vi "MainControlPanel.vi"() -> ()   [LabVIEW 2016]
uses:
  GlobalControlVariables.vi
panel:
  out "Owned":bool
  in  "Acquire Sema":bool
  out "Sema Avail":dbl
  out "Timed Out Sema":bool
  out "Error Messages":string
  in  "QuitVI":bool
  in  "Disconnect":bool
  in  "Chassis Port":u16=8088
  in  "Open Module\n   Controller:":bool
  in  "Module Slot":string(combo)="1"
  out "Connected?":bool
  in  "Connect":bool
  in  "Chassis Address":string="127.0.0.1"
  in  "Module Type":string(combo)="NI-9218"
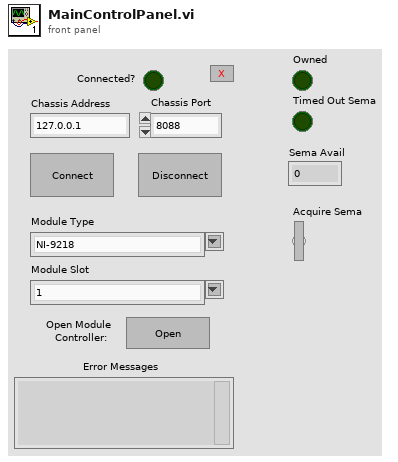
[diagram p1: front panel]
types:
  T1 = typedef "Semaphore RefNum" = refnum<k1>
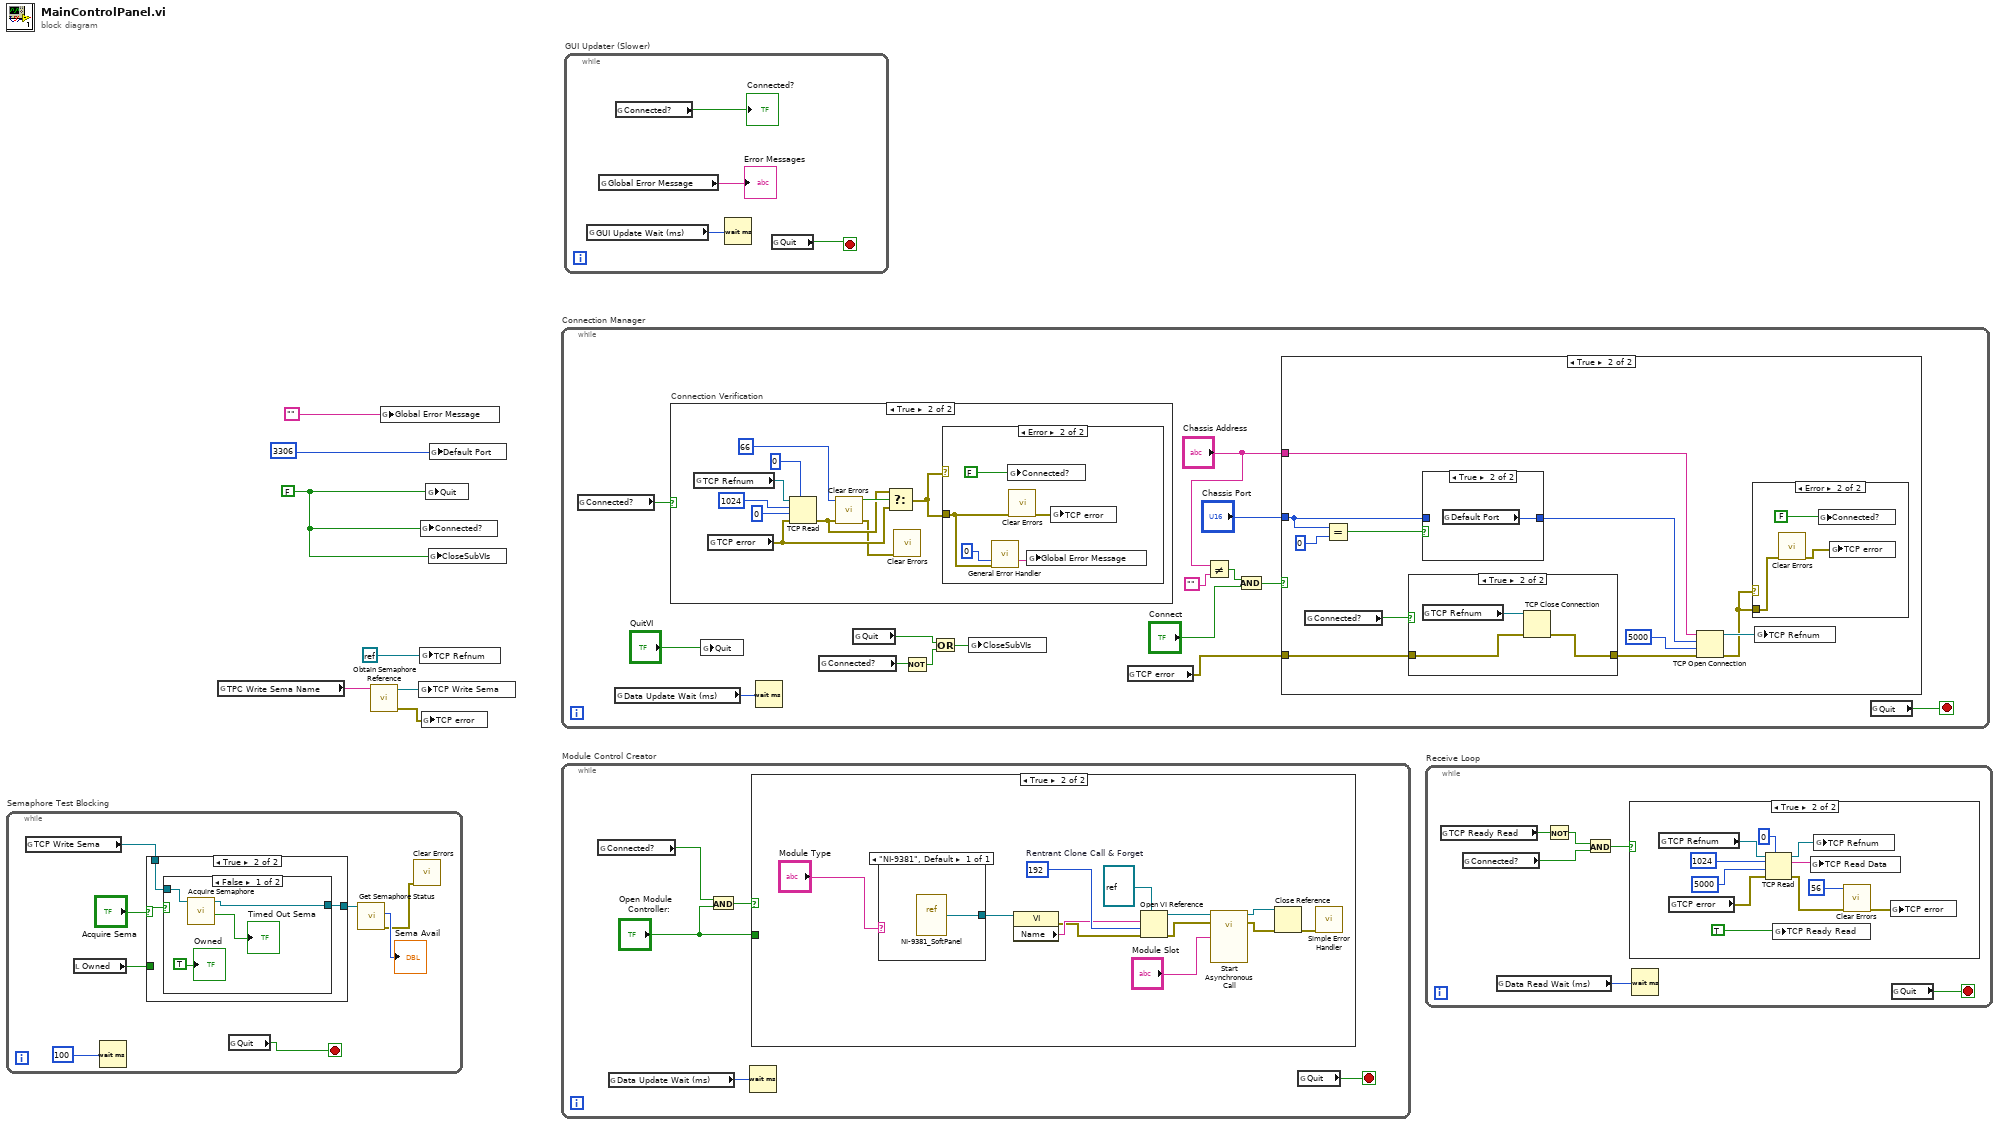
[diagram p0: block diagram]
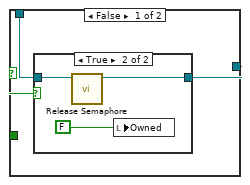
[diagram p2: hidden frame]
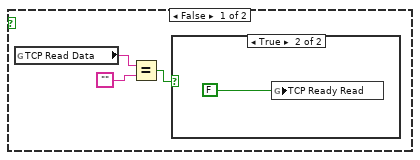
[diagram p5: hidden frame]
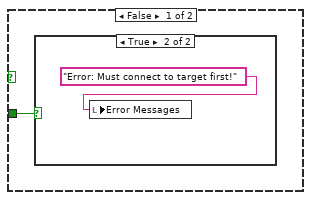
[diagram p7: hidden frame]
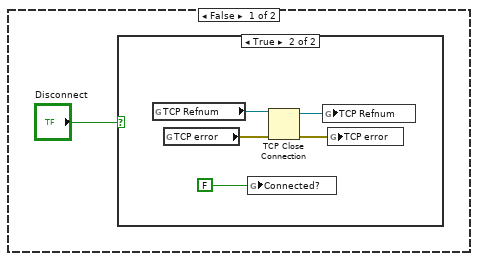
[diagram p11: hidden frame]
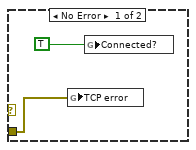
[diagram p13: hidden frame]
diagram:
  w1 = FALSE
  n1 = while "Semaphore Test Blocking" {
    stop <- w14 stop-if-true
    n2 = global read "GlobalControlVariables.vi" "TCP Write Sema"() -> (w9:T1)
    n3 = local read "Owned"() -> (w10:bool)
    n4 = Wait (ms)(milliseconds to wait=u32 100) -> ()  [unwired: 1 out]
    n5 = case shown="True" "Acquire Sema" {
      tunnel: [w18 w25] -> w13
      tunnel: w10 -> [w17 w24]
      tunnel: w9 -> [w16 w23]
      frame False {
        n6 = case shown="True" w17 {
          tunnel: w16 -> [w19 w22]
          tunnel: [w19 w21] -> w18
          frame False {
          }
          frame True {
            n7 = call <vilib>:"Release Semaphore.vi"("semaphore"=w22) -> ("semaphore out"=w21:T1)  [unwired: 5 in, 1 out]
            n8 = local write "Owned"(FALSE) -> ()
          }
        }
      }
      frame True {
        n9 = case shown="False" w24 {
          tunnel: w23 -> [w29 w30]
          tunnel: [w28 w30] -> w25
          frame False {
            n10 = call <vilib>:"Acquire Semaphore.vi"("semaphore"=w29) -> ("timed out"=→"Timed Out Sema":bool, "semaphore out"=w28:T1)  [unwired: 4 in, 1 out]
            "Owned" <- TRUE
          }
          frame True {
          }
        }
      }
    }
    n11 = global read "GlobalControlVariables.vi" "Quit"() -> (w14:bool)
    n12 = call <vilib>:"Get Semaphore Status.vi"("semaphore"=w13) -> ("error out"=w8:errorcluster, "# available"=→"Sema Avail":i32)  [unwired: 5 in, 4 out]
    n13 = call <vilib>:"Clear Errors.vi"("error in (no error)"=w8) -> ()  [unwired: 5 in, 2 out]
  }
  n14 = global read "GlobalControlVariables.vi" "TPC Write Sema Name"() -> (w4:string)
  n15 = call <vilib>:"Obtain Semaphore Reference.vi"("name (unnamed)"=w4) -> ("error out"=w2:errorcluster, "semaphore"=w3:T1)  [unwired: 4 in, 1 out]
  n16 = global write "GlobalControlVariables.vi" "Global Error Message"("") -> ()
  n17 = global write "GlobalControlVariables.vi" "TCP Write Sema"(w3) -> ()
  n18 = global write "GlobalControlVariables.vi" "TCP Refnum"(refnum<k0> refnum) -> ()
  n19 = global write "GlobalControlVariables.vi" "Connected?"(w1) -> ()
  n20 = global write "GlobalControlVariables.vi" "TCP error"(w2) -> ()
  n21 = global write "GlobalControlVariables.vi" "Quit"(w1) -> ()
  n22 = global write "GlobalControlVariables.vi" "CloseSubVIs"(w1) -> ()
  n23 = global write "GlobalControlVariables.vi" "Default Port"(3306) -> ()
  n24 = while "Connection Manager" {
    stop <- w43 stop-if-true
    n25 = global read "GlobalControlVariables.vi" "Connected?"() -> (w42:bool)
    n26 = global read "GlobalControlVariables.vi" "Data Update Wait (ms)"() -> (w36:u32)
    n27 = case "Connection Verification" shown="True" w42 {
      frame False {
      }
      frame True {
        n28 = global read "GlobalControlVariables.vi" "TCP Refnum"() -> (w55:refnum<k5>)
        n29 = global read "GlobalControlVariables.vi" "TCP error"() -> (w49:errorcluster)
        n30 = TCP Read(connection ID=w55, bytes to read=1024, error in (no error)=w49, 7:0, 9:0) -> (error out=w50:errorcluster)  [unwired: 2 out]
        n31 = call <vilib>:"Clear Errors.vi"("error in (no error)"=w50, "specific error code to clear (0: all)"=66) -> ("error out"=w48:errorcluster, "specific error cleared?"=w52:bool)  [unwired: 4 in]
        n32 = Select(t=w50, s=w52, f=w49) -> (s? t:f=w51:errorcluster)
        n33 = call <vilib>:"Clear Errors.vi"("error in (no error)"=w48) -> ()  [unwired: 5 in, 2 out]
        n34 = case shown="Error" w51 {
          tunnel: w51 -> [_ w58]
          frame No Error {
          }
          frame Error {
            n35 = call <vilib>:"General Error Handler.vi"("type of dialog (OK msg:1)"=u16 0, "error in (no error)"=w58) -> ("message"=w56:string)  [unwired: 9 in, 4 out]
            n36 = global write "GlobalControlVariables.vi" "Connected?"(FALSE) -> ()
            n37 = call <vilib>:"Clear Errors.vi"("error in (no error)"=w58) -> ("error out"=w59:errorcluster)  [unwired: 5 in, 1 out]
            n38 = global write "GlobalControlVariables.vi" "Global Error Message"(w56) -> ()
            n39 = global write "GlobalControlVariables.vi" "TCP error"(w59) -> ()
          }
        }
      }
    }
    n40 = global write "GlobalControlVariables.vi" "Quit"("QuitVI") -> ()
    n41 = Wait (ms)(milliseconds to wait=w36) -> ()  [unwired: 1 out]
    n42 = global read "GlobalControlVariables.vi" "Connected?"() -> (w34:bool)
    n43 = global read "GlobalControlVariables.vi" "Quit"() -> (w31:bool)
    n44 = Not(x=w34) -> (.not. x?=w33:bool)
    n45 = Or(x=w31, y=w33) -> (x .or. y?=w32:bool)
    n46 = global write "GlobalControlVariables.vi" "CloseSubVIs"(w32) -> ()
    n47 = global read "GlobalControlVariables.vi" "TCP error"() -> (w35:errorcluster)
    n48 = Not Equal?(x="Chassis Address", y="") -> (x != y?=w39:bool)
    n49 = And(x=w39, y="Connect") -> (x .and. y?=w41:bool)
    n50 = case shown="True" w41 {
      tunnel: "Chassis Port" -> [_ w75]
      tunnel: "Chassis Address" -> [_ w70]
      tunnel: w35 -> [_ w67]
      frame False {
        n51 = case shown="True" "Disconnect" {
          frame False {
          }
          frame True {
            n52 = global read "GlobalControlVariables.vi" "TCP Refnum"() -> (w66:refnum<k5>)
            n53 = global read "GlobalControlVariables.vi" "TCP error"() -> (w65:errorcluster)
            n54 = global write "GlobalControlVariables.vi" "Connected?"(FALSE) -> ()
            n55 = TCP Close Connection(connection ID=w66, error in (no error)=w65) -> (connection ID out=w63:refnum<k5>, error out=w64:errorcluster)  [unwired: 1 in]
            n56 = global write "GlobalControlVariables.vi" "TCP Refnum"(w63) -> ()
            n57 = global write "GlobalControlVariables.vi" "TCP error"(w64) -> ()
          }
        }
      }
      frame True {
        n58 = global read "GlobalControlVariables.vi" "Connected?"() -> (w74:bool)
        n59 = Equal?(x=w75, y=u16 0) -> (x = y?=w76:bool)
        n60 = case shown="True" w74 {
          tunnel: w67 -> [w83 w85]
          tunnel: [w83 w84] -> w72
          frame False {
          }
          frame True {
            n61 = global read "GlobalControlVariables.vi" "TCP Refnum"() -> (w86:refnum<k5>)
            n62 = TCP Close Connection(connection ID=w86, error in (no error)=w85) -> (error out=w84:errorcluster)  [unwired: 1 in, 1 out]
          }
        }
        n63 = case shown="True" w76 {
          tunnel: [w87 w88] -> w71
          tunnel: w75 -> [w87 _]
          frame False {
          }
          frame True {
            n64 = global read "GlobalControlVariables.vi" "Default Port"() -> (w88:u16)
          }
        }
        n65 = TCP Open Connection(address=w70, remote port or service name=w71, timeout ms (60000)=5000, error in (no error)=w72) -> (connection ID=w73:refnum<k5>, error out=w68:errorcluster)  [unwired: 1 in]
        n66 = case shown="Error" w68 {
          tunnel: w68 -> [w78 w80]
          frame No Error {
            n67 = global write "GlobalControlVariables.vi" "TCP error"(w78) -> ()
            n68 = global write "GlobalControlVariables.vi" "Connected?"(TRUE) -> ()
          }
          frame Error {
            n69 = call <vilib>:"Clear Errors.vi"("error in (no error)"=w80) -> ("error out"=w81:errorcluster)  [unwired: 5 in, 1 out]
            n70 = global write "GlobalControlVariables.vi" "Connected?"(FALSE) -> ()
            n71 = global write "GlobalControlVariables.vi" "TCP error"(w81) -> ()
          }
        }
        n72 = global write "GlobalControlVariables.vi" "TCP Refnum"(w73) -> ()
      }
    }
    n73 = global read "GlobalControlVariables.vi" "Quit"() -> (w43:bool)
  }
  n74 = while "Module Control Creator" {
    stop <- w91 stop-if-true
    n75 = global read "GlobalControlVariables.vi" "Connected?"() -> (w93:bool)
    n76 = global read "GlobalControlVariables.vi" "Data Update Wait (ms)"() -> (w89:u32)
    n77 = And(x=w93, y="Open Module\n   Controller:") -> (x .and. y?=w92:bool)
    n78 = Wait (ms)(milliseconds to wait=w89) -> ()  [unwired: 1 out]
    n79 = case shown="True" w92 {
      tunnel: "Open Module\n   Controller:" -> [w94 _]
      frame False {
        n80 = case shown="True" w94 {
          frame False {
          }
          frame True {
            n81 = local write "Error Messages"("Error: Must connect to target first!") -> ()
          }
        }
      }
      frame True {
        w102 = 192  # Rentrant Clone Call & Forget
        n82 = case shown="\"NI-9381\", Default" "Module Type" {
          tunnel: [w108] -> w99
          frame "NI-9381", Default {
            n83 = vi-ref "NI-9381_SoftPanel.vi"() -> (w108:refnum<vi>)
          }
        }
        n84 = property class="VI"(reference=w99) -> (error out=w97:errorcluster, "Name"=w98:string)  [unwired: 1 in, 1 out]
        n85 = Open VI Reference(type specifier VI Refnum (for type only)=refnum<vi> refnum, vi path=w98, options=w102, error in (no error)=w97) -> (vi reference=w101:refnum<vi>, error out=w103:errorcluster)  [unwired: 2 in]
        n86 = call-by-ref "Start Asynchronous Call"(reference=w101, error in=w103, "NI-9381 in Slot:"="Module Slot") -> (reference out=w106:refnum<vi>, error out=w105:errorcluster)  [unwired: 3 in]
        n87 = Close Reference(reference=w106, error in (no error)=w105) -> (error out=w104:errorcluster)
        n88 = call <vilib>:"Simple Error Handler.vi"("error in (no error)"=w104) -> ()  [unwired: 4 in, 5 out]
      }
    }
    n89 = global read "GlobalControlVariables.vi" "Quit"() -> (w91:bool)
  }
  n90 = while "GUI Updater (Slower)" {
    stop <- w110 stop-if-true
    n91 = global read "GlobalControlVariables.vi" "GUI Update Wait (ms)"() -> (w109:u32)
    n92 = global read "GlobalControlVariables.vi" "Global Error Message"() -> (→"Error Messages":string)
    n93 = global read "GlobalControlVariables.vi" "Connected?"() -> (→"Connected?":bool)
    n94 = Wait (ms)(milliseconds to wait=w109) -> ()  [unwired: 1 out]
    n95 = global read "GlobalControlVariables.vi" "Quit"() -> (w110:bool)
  }
  n96 = while "Receive Loop" {
    stop <- w118 stop-if-true
    n97 = global read "GlobalControlVariables.vi" "TCP Ready Read"() -> (w116:bool)
    n98 = global read "GlobalControlVariables.vi" "Connected?"() -> (w114:bool)
    n99 = global read "GlobalControlVariables.vi" "Data Read Wait (ms)"() -> (w113:u32)
    n100 = Not(x=w116) -> (.not. x?=w115:bool)
    n101 = And(x=w115, y=w114) -> (x .and. y?=w117:bool)
    n102 = case shown="True" w117 {
      frame False {
        n103 = global read "GlobalControlVariables.vi" "TCP Read Data"() -> (w120:string)
        n104 = Equal?(x=w120, y="") -> (x = y?=w119:bool)
        n105 = case shown="True" w119 {
          frame False {
          }
          frame True {
            n106 = global write "GlobalControlVariables.vi" "TCP Ready Read"(FALSE) -> ()
          }
        }
      }
      frame True {
        n107 = global read "GlobalControlVariables.vi" "TCP Refnum"() -> (w132:refnum<k5>)
        n108 = global read "GlobalControlVariables.vi" "TCP error"() -> (w131:errorcluster)
        n109 = TCP Read(connection ID=w132, bytes to read=1024, error in (no error)=w131, 7:0, 9:5000) -> (connection ID out=w133:refnum<k5>, data out=w129:string, error out=w124:errorcluster)
        n110 = global write "GlobalControlVariables.vi" "TCP Ready Read"(TRUE) -> ()
        n111 = global write "GlobalControlVariables.vi" "TCP Read Data"(w129) -> ()
        n112 = global write "GlobalControlVariables.vi" "TCP Refnum"(w133) -> ()
        n113 = call <vilib>:"Clear Errors.vi"("error in (no error)"=w124, "specific error code to clear (0: all)"=56) -> ("error out"=w125:errorcluster)  [unwired: 4 in, 1 out]
        n114 = global write "GlobalControlVariables.vi" "TCP error"(w125) -> ()
      }
    }
    n115 = Wait (ms)(milliseconds to wait=w113) -> ()  [unwired: 1 out]
    n116 = global read "GlobalControlVariables.vi" "Quit"() -> (w118:bool)
  }
